vi "Drive_Loop_PID_Update.vi"(10 "PID Gains":T1={"Yaw, Driving Straight"={"proportional gain (Kc)"=1.0, "integral time (Ti, min)"=0.01, "derivative time (Td, min)"=0.0}, "Yaw, Holding Still"={"proportional gain (Kc)"=1.0, "integral time (Ti, min)"=0.01, "derivative time (Td, min)"=0.0}, "Distance, Driving Straight"={"proportional gain (Kc)"=1.0, "integral time (Ti, min)"=0.01, "derivative time (Td, min)"=0.0}, "Distance, Holding Still"={"proportional gain (Kc)"=1.0, "integral time (Ti, min)"=0.01, "derivative time (Td, min)"=0.0}}, 11 "Control Cluster":T2) -> ()   [LabVIEW 2016]
uses:
  <userlib>/836-libraries/Drive/Drive_Code/Drive_Code_Support/Drive_Code_Bundle.ctl
  <userlib>/836-libraries/Drive/Drive_Code/Drive_Code_Support/Sensor_Cluster.ctl
  <userlib>/836-libraries/Drive/Drive_Code/Drive_Code_Support/Camera_Cluster.ctl
  <userlib>/836-libraries/Drive/Drive_Code/Drive_Code_Support/Drive_Code_Notifier.ctl
  <userlib>/836-libraries/Drive/Drive_Code/Drive_Code_Support/Drive_Code_Command.ctl
  <userlib>/836-libraries/Drive/Drive_Code/Logging_Data.ctl
  <userlib>/836-libraries/Drive/Drive_Code/Drive_Code_Support/Drive_Code_PID_Bundle.ctl
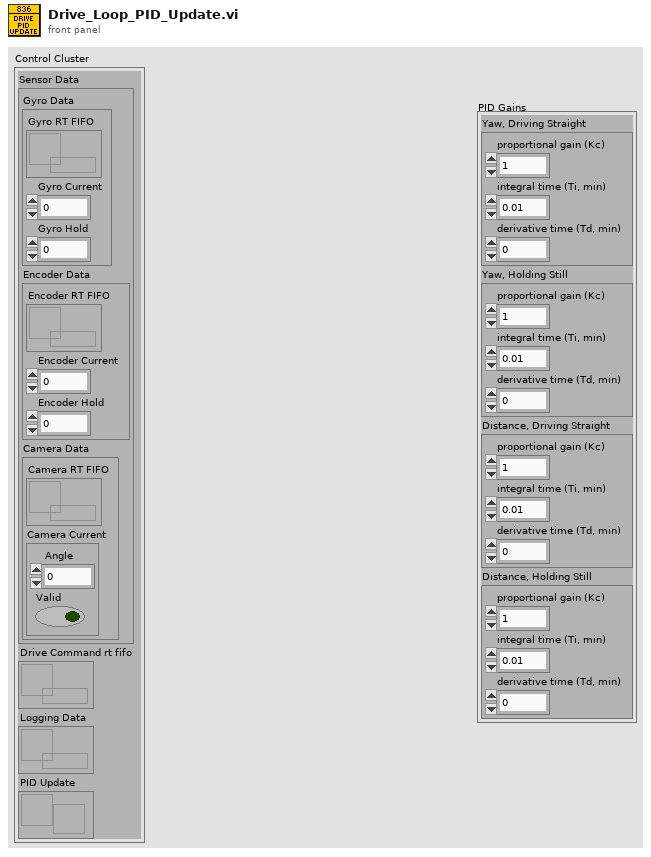
[diagram p1: front panel]
types:
  T1 = typedef "Drive_Code_PID_Bundle.ctl" = cluster{"Yaw, Driving Straight":cluster{"proportional gain (Kc)":dbl, "integral time (Ti, min)":dbl, "derivative time (Td, min)":dbl}, "Yaw, Holding Still":cluster{"proportional gain (Kc)":dbl, "integral time (Ti, min)":dbl, "derivative time (Td, min)":dbl}, "Distance, Driving Straight":cluster{"proportional gain (Kc)":dbl, "integral time (Ti, min)":dbl, "derivative time (Td, min)":dbl}, "Distance, Holding Still":cluster{"proportional gain (Kc)":dbl, "integral time (Ti, min)":dbl, "derivative time (Td, min)":dbl}}
  T2 = typedef "Drive_Code_Bundle.ctl" = cluster{"Sensor Data":T3, "Drive Command rt fifo":refnum<k33>, "Logging Data":refnum<k33>, "PID Update":refnum<notifier>}
  T3 = typedef "Sensor_Cluster.ctl" = cluster{"Gyro Data":cluster{"Gyro RT FIFO":refnum<k33>, "Gyro Current":dbl, "Gyro Hold":dbl}, "Encoder Data":cluster{"Encoder RT FIFO":refnum<k33>, "Encoder Current":dbl, "Encoder Hold":dbl}, "Camera Data":cluster{"Camera RT FIFO":refnum<k33>, "Camera Current":T4}}
  T4 = typedef "Camera_Cluster.ctl" = cluster{" Angle":dbl, "Valid":bool}
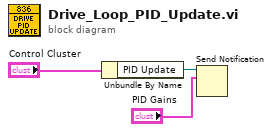
[diagram p0: block diagram]
diagram:
  n1 = Unbundle By Name("Control Cluster") -> ("PID Update"=w2:refnum<notifier>)
  n2 = Send Notification(notification="PID Gains", notifier=w2) -> ()  [unwired: 1 in, 2 out]
